vi "4ChannelSPDTRelay.vi"() -> ()   [LabVIEW 2024]
uses:
  Driver/Public/Digital Pull Direction.ctl
  4d20a38f-85d9-49a3-8b57-4ea18b2081fb.vi
  Driver/CTIPicoVISA.lvlib
panel:
  in  "Load":bool
  out "Switch4LED":bool
  out "Switch3LED":bool
  out "Switch2LED":bool
  out "Switch1LED":bool
  in  "New Address":u8=18 format="%.0x"
  in  "Default Address":u8=17 format="%.0x"
  in  "Stop":bool
  in  "Switch4":bool
  in  "Switch3":bool
  in  "Switch2":bool
  in  "Switch1":bool
  in  "Grove Connector":enum16{"I2C0", "I2C1"}(ring)
  in  "VISA resource name in":refnum<visa-resource-name>="COM15"
  out "Identity":T1
  # "https://wiki.seeedstudio.com/Grove-4-Channel_SPDT_Relay/"
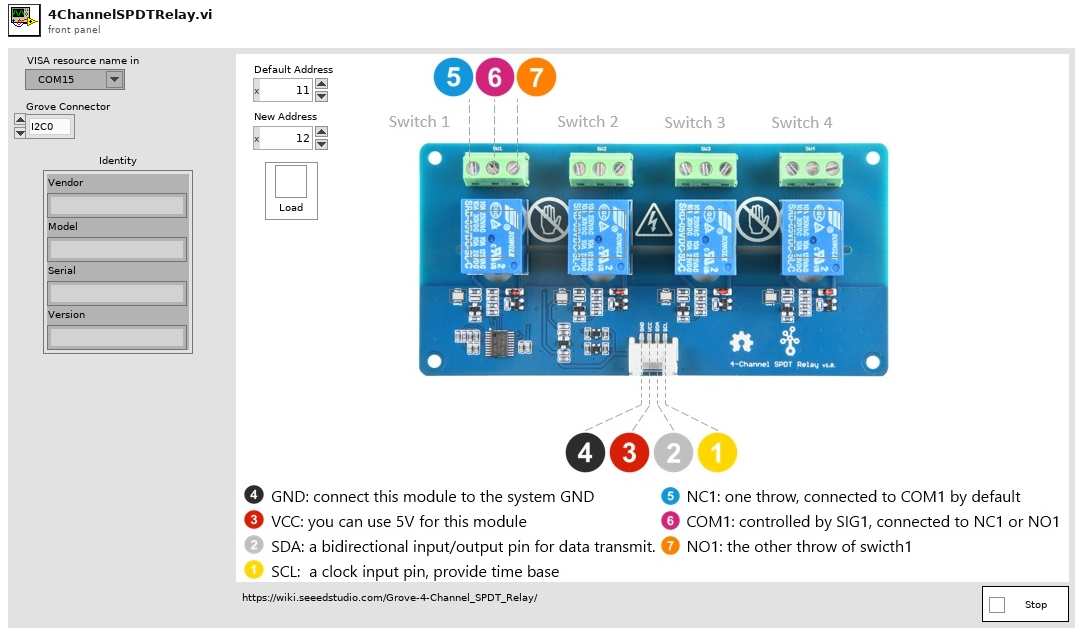
[diagram p1: front panel]
types:
  T1 = cluster{"Vendor":string, "Model":string, "Serial":string, "Version":string}
  T2 = typedef "CTIPicoVISA.lvlib/Digital Pull Direction.ctl" = enum16{"None", "Up", "Down", "Both"}
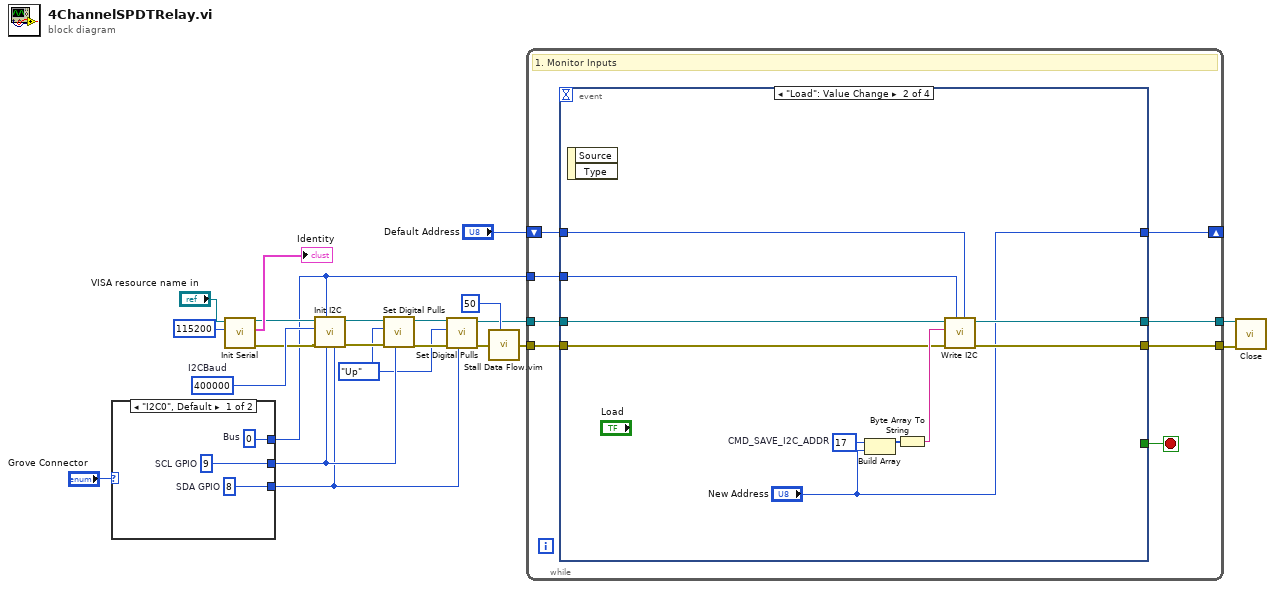
[diagram p0: block diagram]
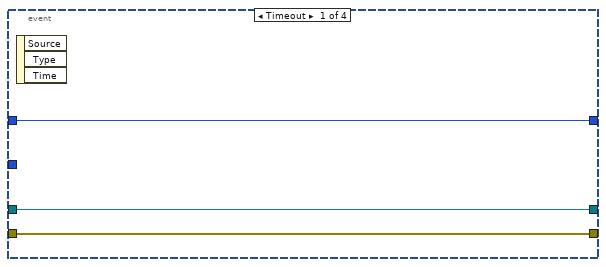
[diagram p2: hidden frame]
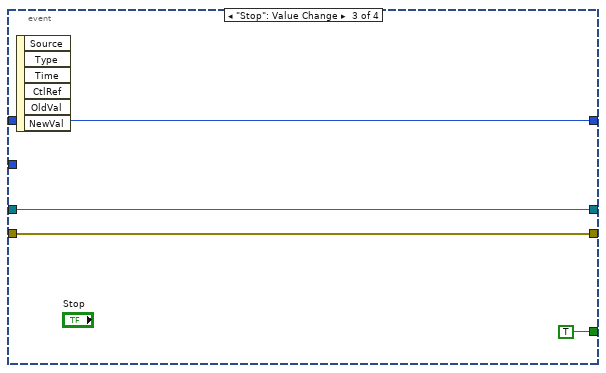
[diagram p3: hidden frame]
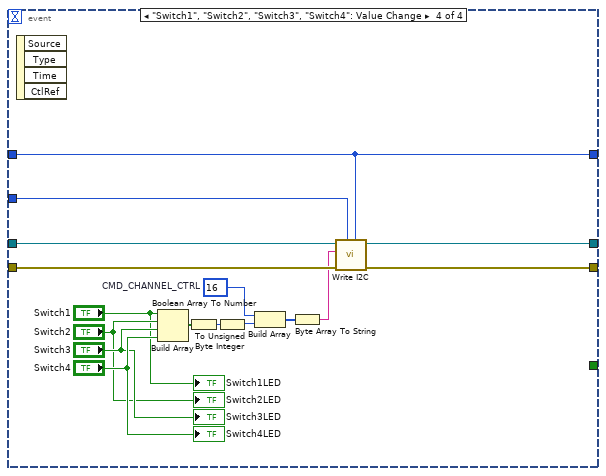
[diagram p4: hidden frame]
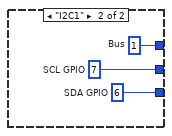
[diagram p5: hidden frame]
diagram:
  w13 = Digital_Pull_Direction."Up" ("Pull")
  w20 = u32 400000  # I2CBaud
  n1 = case shown="\"I2C0\", Default" "Grove Connector" {
    tunnel: [w25 w28] -> w14
    tunnel: [w24 w27] -> w12
    tunnel: [w23 w26] -> w6
    frame "I2C0", Default {
      w23 = u8 0  # Bus
      w24 = 8  # SDA GPIO
      w25 = 9  # SCL GPIO
    }
    frame "I2C1" {
      w26 = u8 1  # Bus
      w27 = 6  # SDA GPIO
      w28 = 7  # SCL GPIO
    }
  }
  n2 = call "Init Serial.vi"("Baud (115200)"=u32 115200, "VISA resource name in"="VISA resource name in") -> ("error out"=w8:errorcluster, "Identity"=→"Identity":T1, "VISA resource name Out"=w9:refnum<visa-resource-name>)  [unwired: 7 in]
  n3 = call "Init I2C.vi"("SDA GPIO"=w12, "SCL GPIO"=w14, "Bus"=w6, "error in (no error)"=w8, "Baud"=w20, "VISA resource name in"=w9) -> ("error out"=w17:errorcluster, "VISA resource name"=w18:refnum<visa-resource-name>)  [unwired: 4 in]
  n4 = call "Set Digital Pulls.vi"("GPIO"=w14, "error in (no error)"=w17, "Pull"=w13, "VISA resource name in"=w18) -> ("error out"=w15:errorcluster, "VISA resource name"=w16:refnum<visa-resource-name>)  [unwired: 6 in]
  n5 = call "Set Digital Pulls.vi"("GPIO"=w12, "error in (no error)"=w15, "Pull"=w13, "VISA resource name in"=w16) -> ("error out"=w10:errorcluster, "VISA resource name"=w1:refnum<visa-resource-name>)  [unwired: 6 in]
  n6 = call "Stall Data Flow.vim"("value in"=w10, "milliseconds to wait"=u32 50) -> ("value out"=w2:errorcluster)  [unwired: 1 out]
  n7 = while {
    tunnel: w6 -> [w31]
    tunnel: w2 -> [w36]
    tunnel: w1 -> [w35]
    tunnel: [w33] -> w3
    tunnel: [w34] -> w4
    shift-right: [w29] -> _
    shift-left: "Default Address" -> [w32]
    stop <- w30 stop-if-true
    # "1. Monitor Inputs"
    n8 = event shown="[1] \"Load\": Value Change" {
      selector: _ -> [_ _ _ _]
      dyn-events: _ -> [_ _ _ _]
      timeout: _ -> [_ _ _ _]
      tunnel: w36 -> [w38 w45 w51 w66]
      tunnel: w35 -> [w39 w46 w52 w67]
      tunnel: [w39 w41 w52 w55] -> w34
      tunnel: [w38 w42 w51 w54] -> w33
      tunnel: w32 -> [w37 w43 w50 w60]
      tunnel: w31 -> [_ w44 _ w61]
      tunnel: [_ _ TRUE ("Stop") _] -> w30
      tunnel: [w37 "New Address" w50 w60] -> w29
      event Timeout {
        n9 = event-data() -> ()  [unwired: 1 in, 3 out]
      }
      event "Load": Value Change {
        w47 = u8 17  # CMD_SAVE_I2C_ADDR
        n10 = event-data() -> ()  [unwired: 1 in, 2 out]
        n11 = Build Array(w47, "New Address") -> (w49:u8[])
        n12 = Byte Array To String(unsigned byte array=w49) -> (string=w48:string)
        n13 = call "Write I2C.vi"("Address"=w43, "Bus"=w44, "error in (no error)"=w45, "Data"=w48, "VISA resource name in"=w46) -> ("error out"=w42:errorcluster, "VISA resource name"=w41:refnum<visa-resource-name>)  [unwired: 5 in]
      }
      event "Stop": Value Change {
        n14 = event-data() -> ()  [unwired: 1 in, 6 out]
      }
      event "Switch1", "Switch2", "Switch3", "Switch4": Value Change {
        w63 = u8 16  # CMD_CHANNEL_CTRL
        n15 = event-data() -> ()  [unwired: 1 in, 4 out]
        n16 = Build Array("Switch1", "Switch2", "Switch3", "Switch4") -> (w68:bool[])
        n17 = Boolean Array To Number(Boolean array=w68) -> (number=w69:u32)
        n18 = To Unsigned Byte Integer(number=w69) -> (unsigned 8bit integer=w65:u8)
        n19 = Build Array(w63, w65) -> (w64:u8[])
        n20 = Byte Array To String(unsigned byte array=w64) -> (string=w62:string)
        n21 = call "Write I2C.vi"("Address"=w60, "Bus"=w61, "error in (no error)"=w66, "Data"=w62, "VISA resource name in"=w67) -> ("error out"=w54:errorcluster, "VISA resource name"=w55:refnum<visa-resource-name>)  [unwired: 5 in]
        "Switch1LED" <- "Switch1"
        "Switch4LED" <- "Switch4"
        "Switch3LED" <- "Switch3"
        "Switch2LED" <- "Switch2"
      }
    }
  }
  n22 = call "Close.vi"("error in (no error)"=w3, "VISA resource name in"=w4) -> ()  [unwired: 9 in, 1 out]
